vi "Send Data with Array SubVI.vi"(0 "Pins In":refnum<k21>[](array[refnum]), 5 "Data":bool[](array[boolean])) -> (6 "Pins Out":refnum<k21>[](array[refnum]))   [LabVIEW 2020]
uses:
  <vilib>/DAQmx/write.llb/DAQmx Write (Digital Bool 1Line 1Point).vi
  <vilib>/DAQmx/miscellaneous.llb/DAQmx Fill In Error Info.vi
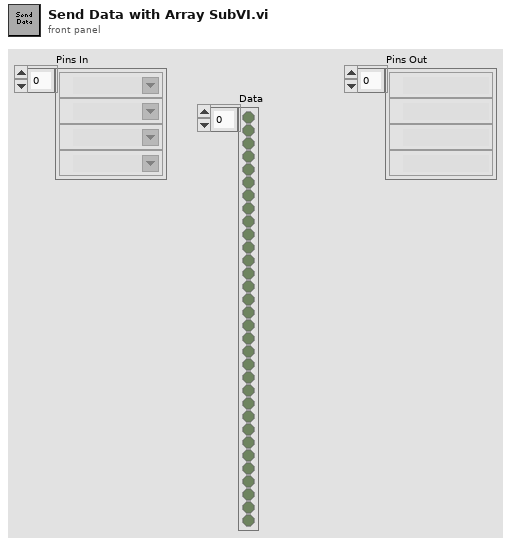
[diagram p1: front panel]
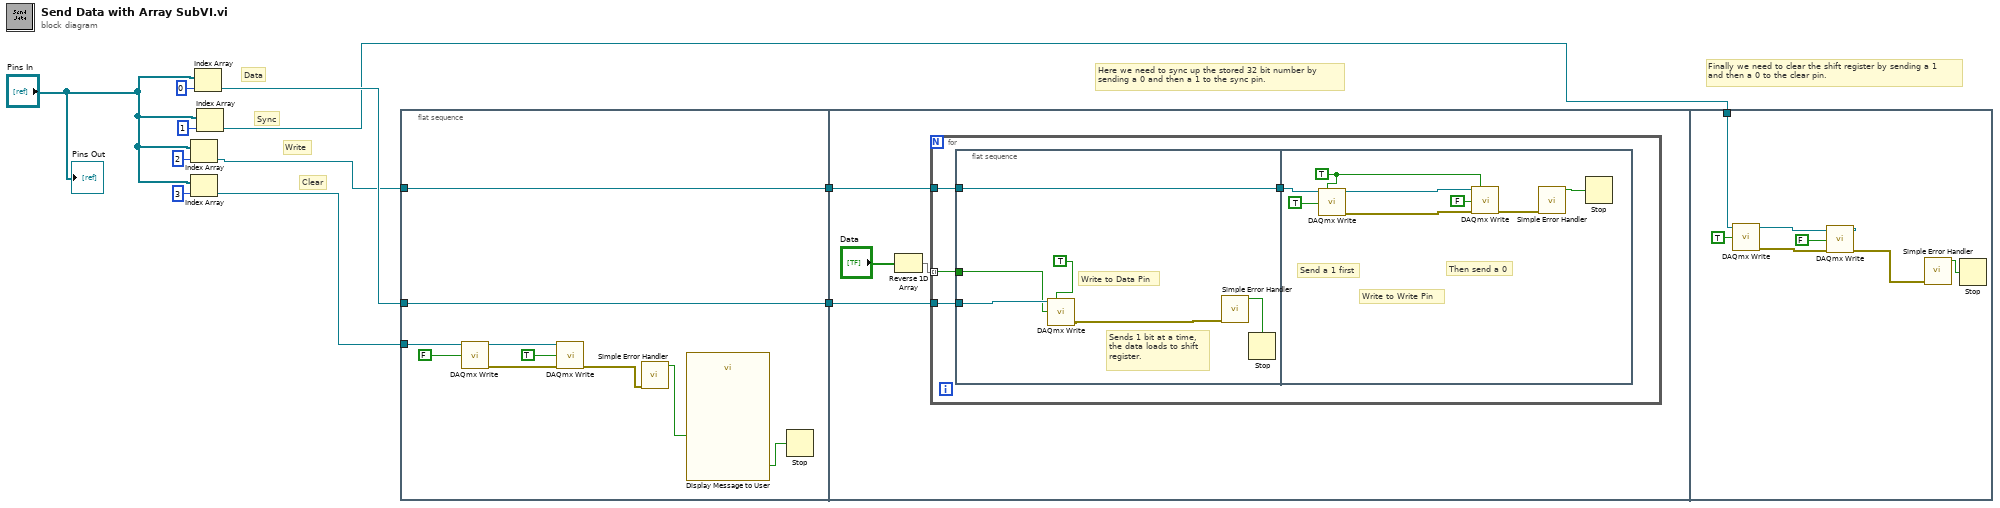
[diagram p0: block diagram]
diagram:
  # "Clear"
  # "Write"
  # "Sync"
  # "Data"
  # "Finally we need to clear the shift register by sending a 1\nand then a 0 to the clear pin."
  # "Here we need to sync up the stored 32 bit number by \nsending a 0 and then a 1 to the sync pin."
  n1 = Index Array(array="Pins In", index=2) -> (element=w3:refnum<k21>)
  n2 = Index Array(array="Pins In", index=3) -> (element=w2:refnum<k21>)
  n3 = Index Array(array="Pins In", index=0) -> (element=w5:refnum<k21>)
  n4 = Index Array(array="Pins In", index=1) -> (element=w4:refnum<k21>)
  n5 = flat-sequence {
    tunnel: w5 -> [w20]
    tunnel: w3 -> [w21]
    tunnel: [w21] -> w11
    tunnel: [w20] -> w10
    tunnel: w2 -> [w14]
    tunnel: w11 -> [w25]
    tunnel: w10 -> [w24]
    tunnel: w4 -> [w45]
    frame #0 {
      n6 = call-poly <vilib>:"DAQmx Write.vi"("task/channels in"=w14, "data"=FALSE) -> ("task out"=w17:refnum<k21>, "error out"=w16:errorcluster)  [unwired: 11 in, 1 out]
      n7 = call-poly <vilib>:"DAQmx Write.vi"("task/channels in"=w17, "data"=TRUE, "error in"=w16) -> ("error out"=w15:errorcluster)  [unwired: 10 in, 2 out]
      n8 = call <vilib>:"Simple Error Handler.vi"("error in (no error)"=w15) -> ("error?"=w13:bool)  [unwired: 4 in, 4 out]
      n9 = call "Display Message to User"("Enable"=w13) -> ("OK"=w12:bool)  [unwired: 9 in, 1 out]
      n10 = Stop(stop? (T)=w12) -> ()
    }
    frame #1 {
      n11 = Reverse 1D Array(array="Data") -> (reversed array=w22:bool[])
      n12 = for {
        tunnel: w25 -> [w29]
        tunnel: w24 -> [w27]
        tunnel: w22 -> [w26] mode=indexing
        n13 = flat-sequence {
          tunnel: w29 -> [w35]
          tunnel: [w35] -> w28
          tunnel: w27 -> [w34]
          tunnel: w26 -> [w33]
          tunnel: w28 -> [w41]
          frame #0 {
            # "Sends 1 bit at a time,\nthe data loads to shift\nregister."
            # "Write to Data Pin"
            n14 = call-poly <vilib>:"DAQmx Write.vi"("task/channels in"=w34, "auto start"=TRUE, "data"=w33) -> ("error out"=w31:errorcluster)  [unwired: 10 in, 2 out]
            n15 = call <vilib>:"Simple Error Handler.vi"("error in (no error)"=w31) -> ("error?"=w30:bool)  [unwired: 4 in, 4 out]
            n16 = Stop(stop? (T)=w30) -> ()
          }
          frame #1 {
            w37 = TRUE
            # "Then send a 0"
            # "Send a 1 first"
            # "Write to Write Pin"
            n17 = call-poly <vilib>:"DAQmx Write.vi"("task/channels in"=w41, "auto start"=w37, "data"=TRUE) -> ("task out"=w38:refnum<k21>, "error out"=w39:errorcluster)  [unwired: 10 in, 1 out]
            n18 = call-poly <vilib>:"DAQmx Write.vi"("task/channels in"=w38, "auto start"=w37, "data"=FALSE, "error in"=w39) -> ("error out"=w40:errorcluster)  [unwired: 9 in, 2 out]
            n19 = call <vilib>:"Simple Error Handler.vi"("error in (no error)"=w40) -> ("error?"=w36:bool)  [unwired: 4 in, 4 out]
            n20 = Stop(stop? (T)=w36) -> ()
          }
        }
      }
    }
    frame #2 {
      n21 = call-poly <vilib>:"DAQmx Write.vi"("task/channels in"=w45, "data"=TRUE) -> ("task out"=w46:refnum<k21>, "error out"=w47:errorcluster)  [unwired: 11 in, 1 out]
      n22 = call-poly <vilib>:"DAQmx Write.vi"("task/channels in"=w46, "data"=FALSE, "error in"=w47) -> ("error out"=w48:errorcluster)  [unwired: 10 in, 2 out]
      n23 = call <vilib>:"Simple Error Handler.vi"("error in (no error)"=w48) -> ("error?"=w44:bool)  [unwired: 4 in, 4 out]
      n24 = Stop(stop? (T)=w44) -> ()
    }
  }
  "Pins Out" <- "Pins In"
